vi "Safe Zone Logic.vi"(9 "Down":bool, 10 "Up":bool, 11 "Limit Switch":bool) -> (3 "Safe Zone":bool)   [LabVIEW 2014]
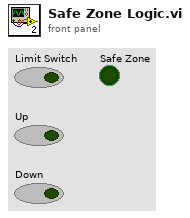
[diagram p1: front panel]
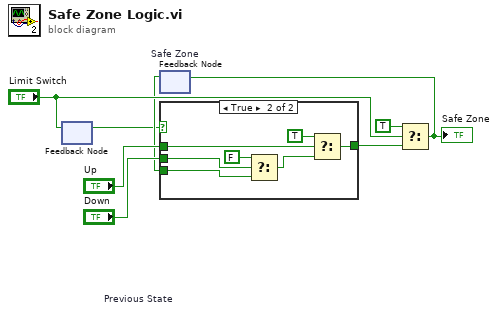
[diagram p0: block diagram]
diagram:
  n1 = feedback #1 "Previous State"() -> (w1:bool)  [unwired: 1 in]
  n2 = feedback-in #1("Limit Switch") -> ()
  n3 = feedback #2 "Safe Zone"() -> (w2:bool)  [unwired: 1 in]
  n4 = case shown="True" w1 {
    tunnel: "Down" -> [_ w16]
    tunnel: w2 -> [w9 w14]
    tunnel: "Up" -> [_ w12]
    tunnel: [w9 w10] -> w4
    frame False {
    }
    frame True {
      n5 = Select(t=FALSE ("Down"), s=w16, f=w14) -> (s? t:f=w13:bool)
      n6 = Select(t=TRUE ("Down"), s=w12, f=w13) -> (s? t:f=w10:bool)
    }
  }
  n7 = Select(t=TRUE, s="Limit Switch", f=w4) -> (s? t:f=w3:bool)
  "Safe Zone" <- w3
  n8 = feedback-in #2(w3) -> ()
